vi "PE Get Wavelength.vi"(8 "error in (no error)":errorcluster, 11 "peHandle":u32) -> (0 "error out":errorcluster, 2 "function return":i32, 3 "wavelength":dbl)   [LabVIEW 2011, in "libPhyspec.lvlib"]
doc: "PHYSPEC_API PE_STATUS PE_GetWavelength(CPE_HANDLE peHandle, double *wavelength);"
uses:
  libPhyspec.lvlib
  libPhyspec.dll
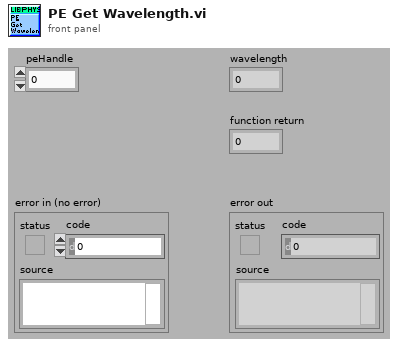
[diagram p1: front panel]
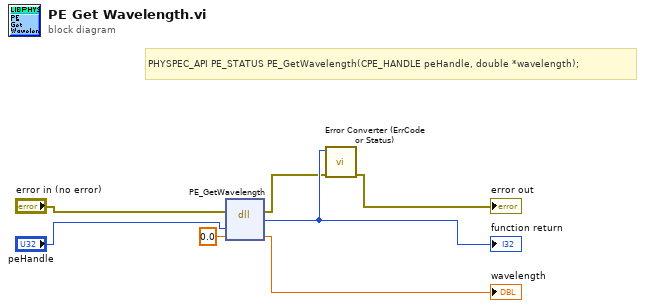
[diagram p0: block diagram]
diagram:
  # "PHYSPEC_API PE_STATUS PE_GetWavelength(CPE_HANDLE peHandle, double *wavelength);"
  n1 = dll-call lib="D:/users/nicolas/PHySpec-SDK-1.0.0/Labview-example/libPhyspec/libPhyspec.*" fn="PE_GetWavelength"(error in="error in (no error)", "peHandle"="peHandle", "wavelength"=0.0) -> (error out=w2:errorcluster, w7:i32, "wavelength"=→"wavelength":dbl)  [unwired: 3 in, 1 out]
  "function return" <- w7
  n2 = call "Error Converter (ErrCode or Status).vi"("error in (no error)"=w2, "error code"=w7) -> ("error out"=→"error out":errorcluster)  [unwired: 9 in]
